vi "gfitsio-read-image-subset-dbl-3d.vi"(4 "lpixel (-1,-1,-1: rest)":cluster{"X":i32, "Y":i32, "Z":i32}={"X"=-1, "Y"=-1, "Z"=-1}, 6 "fpixel (1,1,1)":cluster{"X":i32, "Y":i32, "Z":i32}={"X"=1, "Y"=1, "Z"=1}, 7 "inc (1,1,1)":cluster{"X":i32, "Y":i32, "Z":i32}={"X"=1, "Y"=1, "Z"=1}, 8 "error in (no error)":errorcluster, 9 "nulval (0: don't check)":dbl, 11 "gfits refnum":T1) -> (0 "error out":errorcluster, 1 "anynul":bool, 2 "data":dbl[][][](array[numeric]), 3 "dup gfits refnum":T1)   [LabVIEW 2019, in "gfitsio.lvlib"]
doc: "Read a rectangular subimage (or the whole image) from the FITS data array. <B>fpixel</B> and <B>lpixel</B> give the coordinates of the first (lower left corner) and last (upper right corner) pixels to be read from the FITS image. Undefined FITS array elements will be set equal to <B>nullval</B> unless <B>nulval</B> is zero in which case no checks for undefined pixels will be performed."
uses:
  gfitsio.lvlib
  gfitsio-refnum.ctl
  cfitsio-hdutypes.ctl
  gfitsio.dll
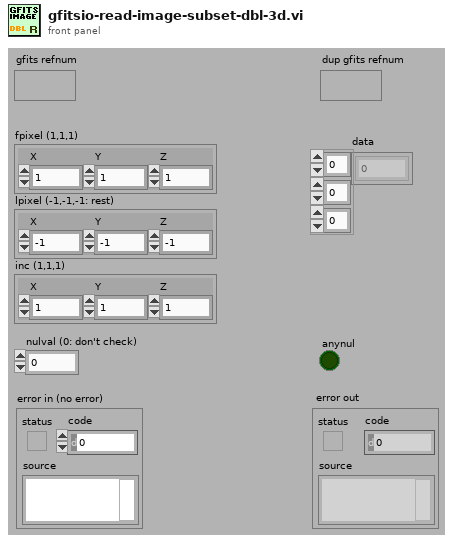
[diagram p1: front panel]
types:
  T1 = typedef "gfitsio.lvlib/gfitsio-refnum.ctl" = refnum<k1>
  T2 = typedef "gfitsio.lvlib/cfitsio-hdutypes.ctl" = i32
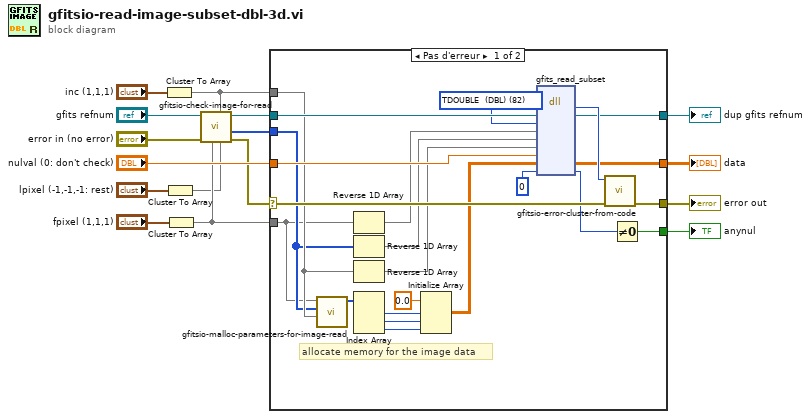
[diagram p0: block diagram]
diagram:
  n1 = Cluster To Array(cluster="inc (1,1,1)") -> (array=w1:i32[])
  n2 = Cluster To Array(cluster="lpixel (-1,-1,-1: rest)") -> (array=w2:i32[])
  n3 = Cluster To Array(cluster="fpixel (1,1,1)") -> (array=w3:i32[])
  n4 = call "gfitsio-check-image-for-read.vi"("lpixel"=w2, "inc"=w1, "fpixel"=w3, "error in (no error)"="error in (no error)", "gfits refnum"="gfits refnum") -> ("error out"=w5:errorcluster, "lpixel out"=w4:i32[], "dup gfits refnum"=w10:T1)  [unwired: 4 in]
  n5 = case shown="Pas d'erreur" w5 {
    selector: w5 -> [w34 w40]
    tunnel: [w38 w40] -> w15
    tunnel: w10 -> [w36 w41]
    tunnel: [w35 w41] -> w16
    tunnel: "nulval (0: don't check)" -> [w33 _]
    tunnel: [w31 _] -> w13
    tunnel: [w30 _] -> w12
    tunnel: w3 -> [w23 _]
    tunnel: w4 -> [w24 _]
    tunnel: w1 -> [w25 _]
    frame No Error {
      w29 = T2 82 items=["TBIT"=1, "TBYTE  (U8)"=11, "TSBYTE  (I8)"=12, "TLOGICAL"=14, "TSTRING"=16, "TUSHORT  (U16)"=20, "TSHORT  (I16)"=21, "TUINT"=31, "TULONG  (U32)"=40, "TLONG  (I32)"=41, "TFLOAT  (SGL)"=42, "TLONGLONG  (I64)"=81, "TDOUBLE  (DBL)"=82, "TCOMPLEX  (CSG)"=83, "TDOUBLECOMPLEX  (CDB)"=163] ("cfitsio datatype")
      # "allocate memory for the image data"
      n6 = call "gfitsio-malloc-parameters-for-image-read.vi"("inc"=w25, "lpixel"=w24, "fpixel"=w23) -> ("image dimensions"=w20:i32[])  [unwired: 8 in]
      n7 = Reverse 1D Array(array=w23) -> (reversed array=w26:i32[])
      n8 = Reverse 1D Array(array=w24) -> (reversed array=w27:i32[])
      n9 = Reverse 1D Array(array=w25) -> (reversed array=w28:i32[])
      n10 = Index Array(array=w20) -> (element #1=w19:i32, element #2=w18:i32, element #3=w17:i32)  [unwired: 3 in]
      n11 = Initialize Array(0.0 ("element"), w19, w18, w17) -> (w21:dbl[][][])
      n12 = dll-call lib="C:/BonOMM_git/SubVIs/gfitsio/gfitsio.dll" fn="gfits_read_subset"("dup gfits refnum"=w36, "datatype"=w29, "fpixel"=w26, "lpixel"=w27, "inc"=w28, "nulval"=w33, "array"=w21, "anynul"=0) -> (w39:i32, "dup gfits refnum"=w35:T1, "array"=w30:dbl[][][], "anynul"=w32:i32)  [unwired: 8 in, 2 out]
      n13 = call "gfitsio-error-cluster-from-code.vi"("error in (no error)"=w34, "error code"=w39) -> ("error out"=w38:errorcluster)  [unwired: 9 in]
      n14 = Not Equal To 0?(x=w32) -> (x != 0?=w31:bool)
    }
    frame Error {
    }
  }
  "dup gfits refnum" <- w16
  "error out" <- w15
  "anynul" <- w13
  "data" <- w12
